vi "Render.vi"(8 "error in (no error)":errorcluster, 10 "String in":string, 11 "Collection in":refnum<class "Collection.lvclass">) -> (0 "error out":errorcluster, 2 "String out":string, 3 "Collection out":refnum<class "Collection.lvclass">)   [LabVIEW 2021, in "Markdown.lvlib" / "Collection.lvclass"]
uses:
  Collection.lvclass
  Collection.lvclass/Collection.ctl
  IRenderable/IRenderable.lvclass
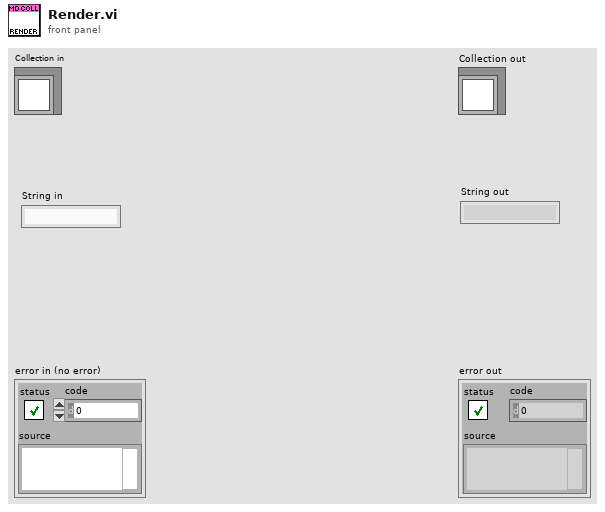
[diagram p1: front panel]
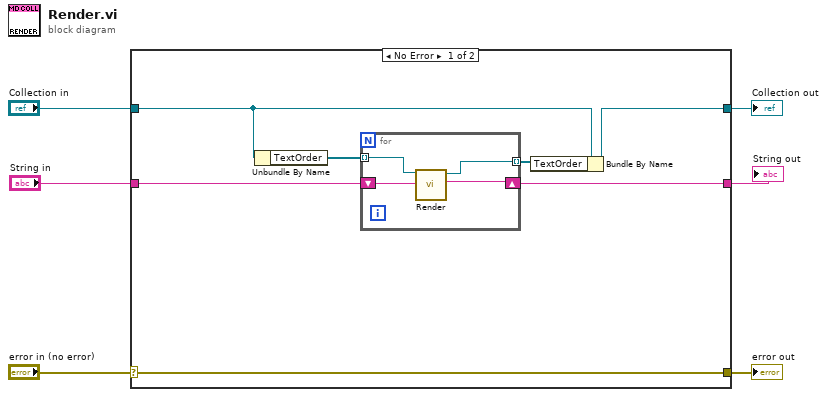
[diagram p0: block diagram]
diagram:
  n1 = case shown="No Error" "error in (no error)" {
    selector: "error in (no error)" -> [w13 w20]
    tunnel: [w13 w20] -> w5
    tunnel: [w9 w19] -> w3
    tunnel: "Collection in" -> [w8 w19]
    tunnel: "String in" -> [w12 w18]
    tunnel: [w7 w18] -> w1
    frame No Error {
      n2 = Unbundle By Name(w8) -> ("TextOrder"=w11:refnum<class "IRenderable.lvclass">[])
      n3 = for {
        tunnel: w11 -> [w16] mode=indexing
        tunnel: [w15] -> w10 mode=indexing
        shift-right: [w14] -> w7
        shift-left: w12 -> [w17]
        n4 = call-dynamic "Render.vi"("String in"=w17, "IRenderable in"=w16) -> ("String out"=w14:string, "IRenderable out"=w15:refnum<class "IRenderable.lvclass">)  [unwired: 7 in, 1 out]
      }
      n5 = Bundle By Name(cluster=w8, "TextOrder"=w10) -> (w9:refnum<class "Collection.lvclass">)
    }
    frame Error {
    }
  }
  "error out" <- w5
  "Collection out" <- w3
  "String out" <- w1
